vi "Comm_mult_tcp2.vi"(11 "ConfigFile":path=path "/home/ArcVIEW/Modules/TCSP60/config/TCSP60_Default.cfg") -> ()   [LabVIEW 2016]
doc: "Main VI for the COMSTCP Module. This module is in charge of the externl TCP/IP comunications"
panel:
  in  "openpanel":bool
  out "last async.":string
  in  "async_on_block":bool
  in  "cmdset":string="NATIVE"
  out "async port":u16
  out "async":refnum<k5>
  out "last response":string
  out "last command":string
  out "error out 2":errorcluster
  out "block_port":u16=1502
  in  "blockport":u16
  in  "maxasyncinst":i8=2
  in  "maxcmdinst":i8=2
  in  "asyncport":u16=1320
  out "cmd listener ID":refnum<k5>
  in  "Log":bool
  in  "logfile":path
  out "cmd port":u16
  out "error out":errorcluster
  in  "cmdport":u16=1320
  in  "Initialization Variables":string[][](table)=[["mult_tcp2", "asyncport", "Comm_mult_tcp2.vi", "asyncport", "1501", "U16"], ["mult_tcp2", "multport", "Comm_mult_tcp2.vi", "cmdport", "1500", "U16"], ["mult_tcp2", "cmdport", "Comm_mult_tcp2.vi", "blockport", "1502", "U16"], ["mult_tcp2", "maxcmdsvr", "Comm_mult_tcp2.vi", "maxcmdinst", "", "I8"], ["mult_tcp2", "maxasyncsvr", "Comm_mult_tcp2.vi", "maxasyncinst", "", "I8"], ["mult_tcp2", "log", "Comm_mult_tcp2.vi", "Log", "yes", "BOOL"], ["mult_tcp2", "file", "Comm_mult_tcp2.vi", "logfile", "", "PATH"], ["mult_tcp2", "cmdset", "Comm_mult_tcp2.vi", "cmdset", "", "STR"], ["mult_tcp2", "asynconblock", "Comm_mult_tcp2.vi", "async_on_block", "", "BOOL"], ["mult_tcp2", "openpanel", "Comm_mult_tcp2.vi", "openpanel", "", "BOOL"]]
  in  "error in":errorcluster
  in  "ModuleName":string="MULTTCP2"
  out "stopped":bool=TRUE
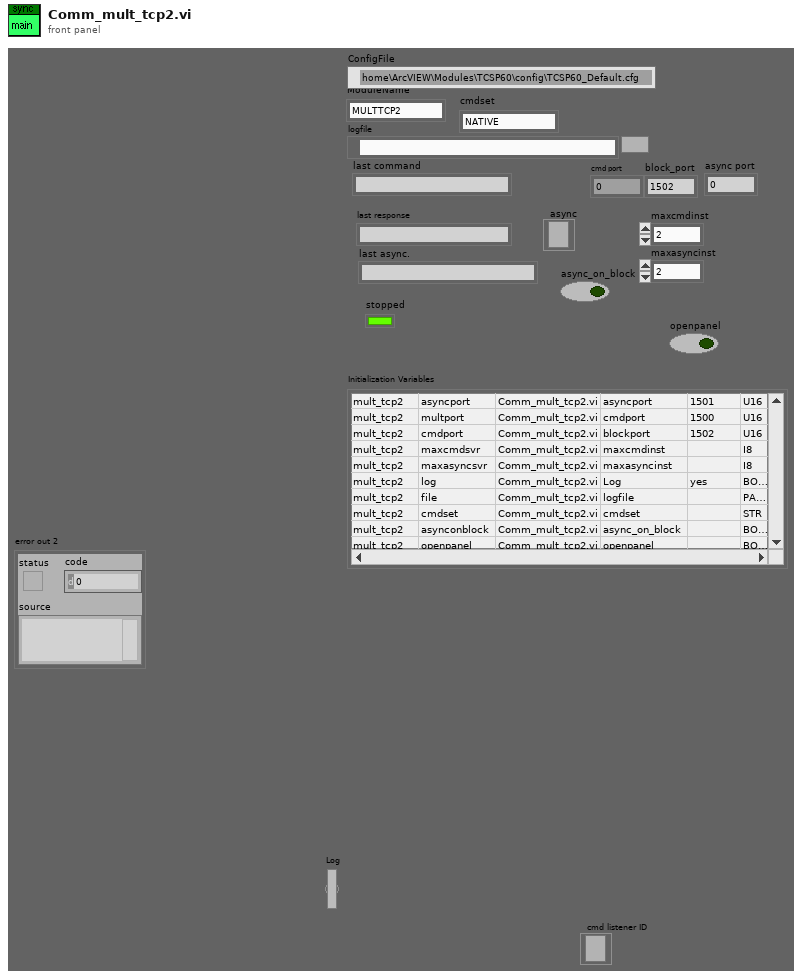
[diagram p1: front panel]
types:
  T1 = cluster{"t":string, "blockport":u16, "cmdport":u16, "asyncport":u16}
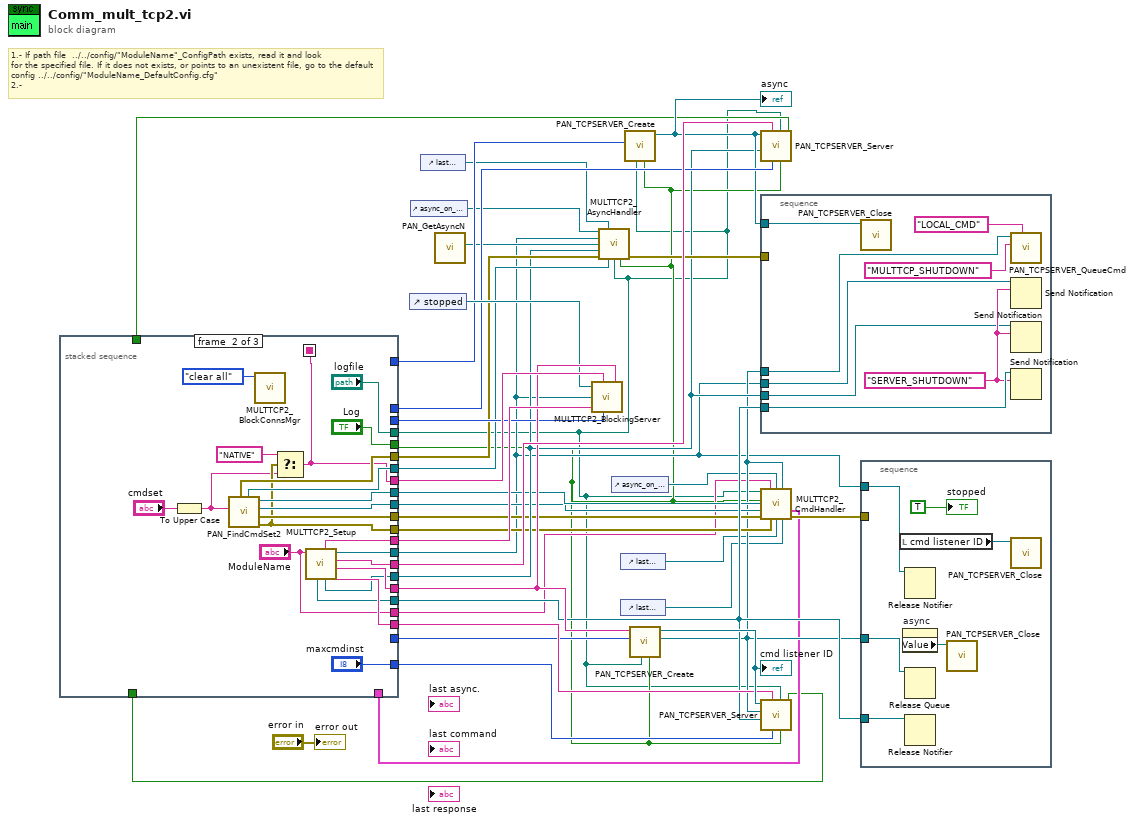
[diagram p0: block diagram]
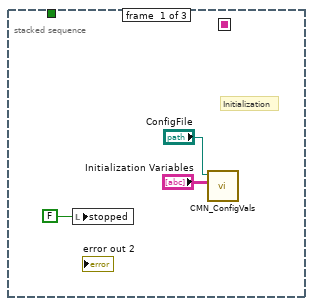
[diagram p2: hidden frame]
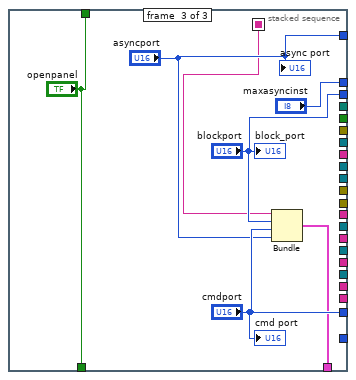
[diagram p3: hidden frame]
diagram:
  # "1.- If path file  ../../config/\"ModuleName\"_ConfigPath exists, read it and look\nfor the specified file. If it does not exists, or points to an unexistent file, go to the default\nconfig ../../config/\"ModuleName_DefaultConfig.cfg\"\n2.-"
  n1 = stacked-sequence {
    seq-local: [_ w42 _] -> [_ _ w66]
    tunnel: [_ w48 _] -> w19
    tunnel: [_ "maxcmdinst" _] -> w37
    tunnel: [_ w52 _] -> w8
    tunnel: [_ w47 _] -> w25
    tunnel: [_ w61 _] -> w17
    tunnel: [_ w60 _] -> w15
    tunnel: [_ w59 _] -> w16
    tunnel: [_ w55 _] -> w14
    tunnel: [_ w58 _] -> w22
    tunnel: [_ w57 _] -> w24
    tunnel: [_ w50 _] -> w32
    tunnel: [_ w51 _] -> w36
    tunnel: [_ w49 _] -> w35
    tunnel: [_ w42 _] -> w34
    tunnel: [_ w46 _] -> w33
    tunnel: [_ _ "asyncport"] -> w30
    tunnel: [_ _ "maxasyncinst"] -> w29
    tunnel: [_ _ "cmdport"] -> w28
    tunnel: [_ _ "blockport"] -> w27
    tunnel: [_ "logfile" _] -> w1
    tunnel: [_ "Log" _] -> w2
    tunnel: [_ "ModuleName" _] -> w6
    tunnel: [_ _ w65] -> w5
    tunnel: [_ _ "openpanel"] -> w4
    tunnel: [_ _ "openpanel"] -> w3
    frame #0 {
      # "Initialization"
      n2 = local write "stopped"(FALSE ("stopped")) -> ()
      n3 = call "CMN_ConfigVals.vi"("ConfigVariables"="Initialization Variables", "configuration file path"="ConfigFile") -> ()  [unwired: 2 in, 8 out]
    }
    frame #1 {
      n4 = To Upper Case(1:"cmdset") -> (0:w53:string)
      n5 = call "PAN_FindCmdSet2.vi"("cmdset"=w53) -> ("error resp out"=w55:errorcluster, "error cmd out"=w60:errorcluster, "respref"=w59:refnum<vi>, "cmdref"=w61:refnum<vi>, "async reference"=w58:refnum<vi>, "error async out"=w57:errorcluster)  [unwired: 5 out]
      n6 = call "MULTTCP2_BlockConnsMgr.vi"("action"=enum16{"add", "delete", "find", "clear all"}."clear all") -> ()  [unwired: 3 in, 8 out]
      n7 = Select(t="NATIVE", s=w55, f=w53) -> (s? t:f=w42:string)
      n8 = call "MULTTCP2_Setup.vi"("module name"="ModuleName") -> ("multcmd1"=w49:string, "cmdq"=w50:string, "async notifier name"=w51:string, "block notifier"=w52:refnum<notifier>, "async notifier"=w48:refnum<notifier>, "blockID"=w46:string, "cmd notif"=w47:refnum<notifier>)  [unwired: 4 out]
    }
    frame #2 {
      n9 = Bundle("t"=w66, "blockport"="blockport", "cmdport"="cmdport", "asyncport"="asyncport") -> (w65:T1)  [unwired: 1 out]
      "async port" <- "asyncport"
      "cmd port" <- "cmdport"
      "block_port" <- "blockport"
    }
  }
  n10 = control-ref of="stopped"() -> (w31:refnum<vi>)
  n11 = control-ref of="async_on_block"() -> (w7:refnum<vi>)
  n12 = control-ref of="last async."() -> (w18:refnum<vi>)
  n13 = call "PAN_GetAsyncN.vi"() -> ("asyncN"=w23:refnum<notifier>)  [unwired: 11 out]
  n14 = call "MULTTCP2_BlockingServer.vi"("stot ref"=w31, "cmdset"=w34, "block notifier"=w8, "blockID"=w33, "blockport"=w27, "cmdq"=w32) -> ()
  n15 = call "MULTTCP2_AsyncHandler.vi"("async_on_block"=w7, "last async ref"=w18, "block notifier"=w8, "asyncN"=w23, "async notifier"=w19, "error async out"=w24, "async reference"=w22, "logfile"=w1, "Log"=w2) -> ("error async out"=w20:errorcluster)  [unwired: 6 out]
  n16 = control-ref of="async_on_block"() -> (w11:refnum<vi>)
  n17 = control-ref of="last command"() -> (w9:refnum<vi>)
  n18 = control-ref of="last response"() -> (w10:refnum<vi>)
  n19 = call "PAN_TCPSERVER_Create.vi"("log"=w2, "logfile"=w1, "port"=w30) -> ("listener ID"=w21:refnum<k5>)  [unwired: 2 in, 6 out]
  "async" <- w21
  n20 = call "PAN_TCPSERVER_Create.vi"("log"=w2, "logfile"=w1, "port"=w28, "messages from socks Q name"=w32) -> ("queue out"=w13:refnum<queue>, "listener ID"=w38:refnum<k5>)  [unwired: 1 in, 5 out]
  "cmd listener ID" <- w38
  n21 = call "PAN_TCPSERVER_Server.vi"("open panel"=w4, "log"=w2, "logfile"=w1, "max instances"=w29, "callerID"=w36, "notifier In"=w19, "listener ID"=w21) -> ()  [unwired: 1 in, 4 out]
  n22 = stacked-sequence {
    tunnel: w25 -> [w78]
    tunnel: w8 -> [w77]
    tunnel: w13 -> [w73]
    tunnel: w21 -> [w72]
    tunnel: w20 -> [_]
    tunnel: w19 -> [w71]
    frame #0 {
      w76 = "SERVER_SHUTDOWN" ("notification")
      n23 = call "PAN_TCPSERVER_Close.vi"("listener ID"=w72) -> ()  [unwired: 1 in, 10 out]
      n24 = call "PAN_TCPSERVER_QueueCmd.vi"("ID"="LOCAL_CMD", "command"="MULTTCP_SHUTDOWN", "queue in"=w73) -> ()  [unwired: 3 in, 6 out]
      n25 = Send Notification(notification=w76, notifier=w77) -> ()  [unwired: 1 in, 2 out]
      n26 = Send Notification(notification=w76, notifier=w71) -> ()  [unwired: 1 in, 2 out]
      n27 = Send Notification(notification=w76, notifier=w78) -> ()  [unwired: 1 in, 2 out]
    }
  }
  n28 = call "MULTTCP2_CmdHandler.vi"("logfile"=w1, "taskID"=w6, "async on block"=w11, "cmd queue"=w13, "Log"=w2, "cmdref"=w17, "respref"=w16, "info cluster"=w5, "error cmd out"=w15, "error resp out"=w14, "last cmd"=w9, "last response"=w10) -> ("error resp out"=w12:errorcluster)  [unwired: 3 out]
  n29 = call "PAN_TCPSERVER_Server.vi"("open panel"=w3, "log"=w2, "logfile"=w1, "max instances"=w37, "callerID"=w35, "notifier In"=w25, "messages from sock"=w13, "listener ID"=w38) -> ()  [unwired: 4 out]
  n30 = stacked-sequence {
    tunnel: w25 -> [w83]
    tunnel: w8 -> [w82]
    tunnel: w13 -> [w79]
    tunnel: w12 -> [_]
    frame #0 {
      n31 = local read "cmd listener ID"() -> (w80:refnum<k5>)
      n32 = property on="async" class="Ref (strict)"() -> ("Value"=w81:refnum<k5>)  [unwired: 2 in, 2 out]
      n33 = Release Notifier(notifier=w82) -> ()  [unwired: 1 in, 4 out]
      n34 = Release Queue(queue=w79) -> ()  [unwired: 1 in, 4 out]
      n35 = Release Notifier(notifier=w83) -> ()  [unwired: 1 in, 4 out]
      n36 = call "PAN_TCPSERVER_Close.vi"("listener ID"=w81) -> ()  [unwired: 1 in, 10 out]
      n37 = call "PAN_TCPSERVER_Close.vi"("listener ID"=w80) -> ()  [unwired: 1 in, 10 out]
      "stopped" <- TRUE
    }
  }
  "error out" <- "error in"
